vi "Part 2.vi"(11 "Input":string) -> (3 "Output":i64)   [LabVIEW 2021]
uses:
  <vilib>/Utility/miscctls.llb/LVMapReplaceAction.ctl
  2fdae834-c3bc-4fab-b255-983e670ed845.vi
  e0cb1816-1f8c-444e-8856-724e2788fbe8.vi
  <userlib>/_OpenG.lib/string/string.llb/Convert EOLs (String)__ogtk.vi
  <vilib>/Comparison/Equal/Equal Functor/Equal Functor.lvclass
panel:
  out "array":string[](array[string])
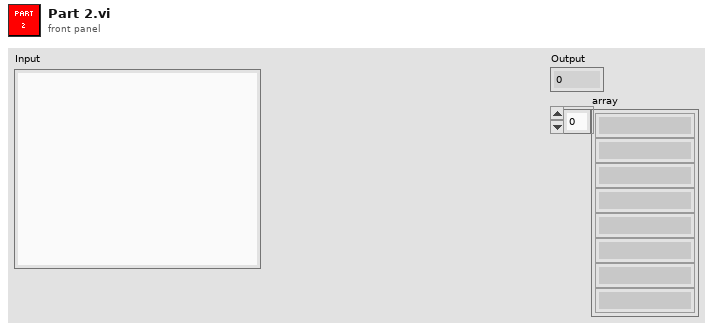
[diagram p1: front panel]
types:
  T1 = map{i32, cluster{"Lens":string[], "Focal Length":i32[]}}
  T2 = typedef "LVMapReplaceAction.ctl" = enum32{"Modify Entry only if found", "Add or Modify Entry", "Delete Entry"}
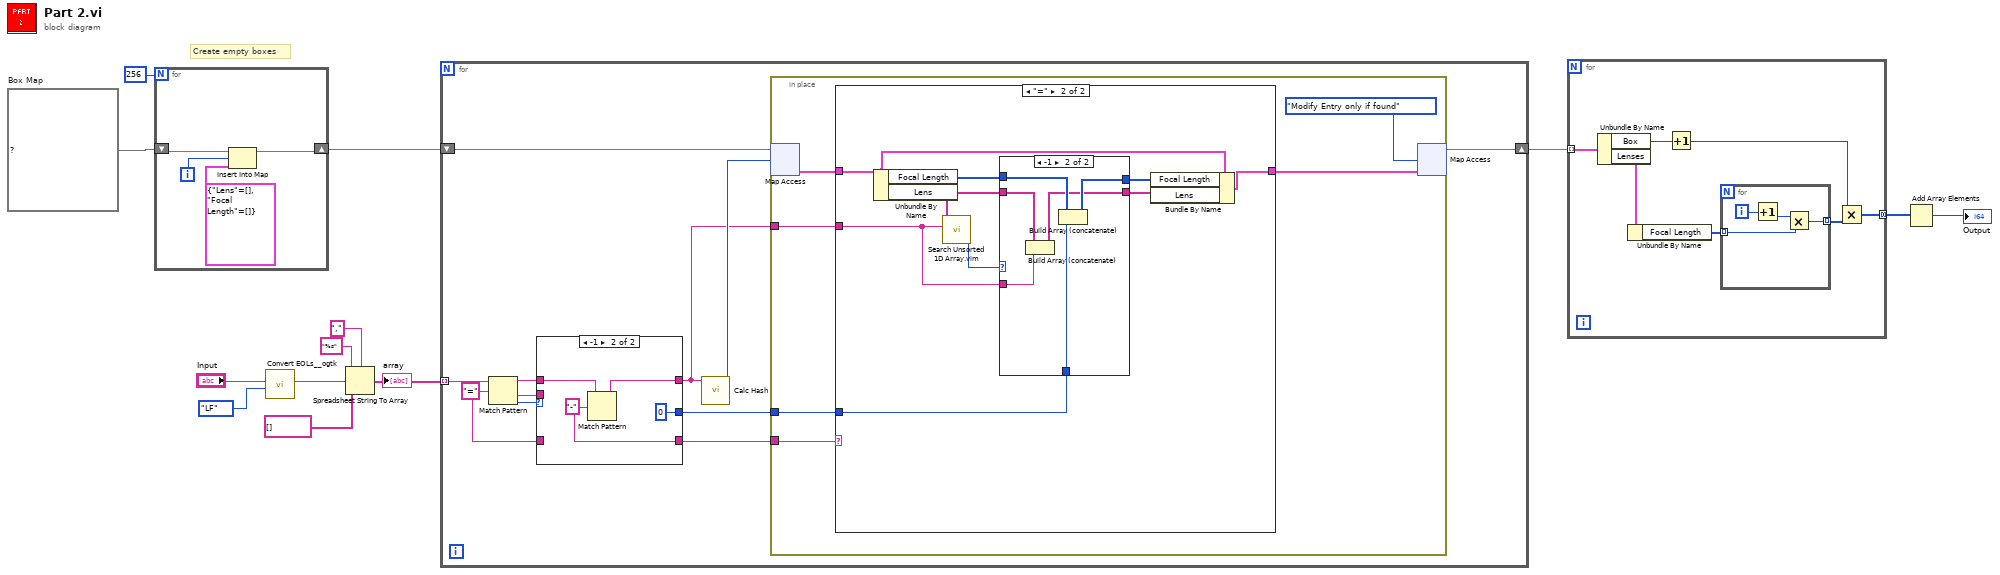
[diagram p0: block diagram]
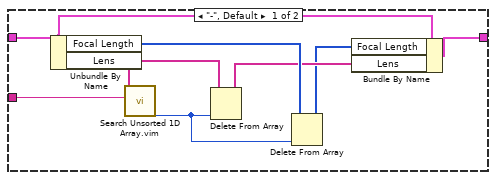
[diagram p2: hidden frame]
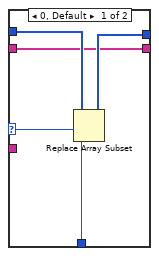
[diagram p3: hidden frame]
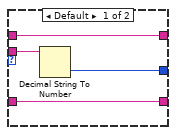
[diagram p4: hidden frame]
diagram:
  w6 = T1 {}  # Box Map
  # "Create empty boxes"
  n1 = for {
    N: 256 -> [_]
    shift-right: [w16] -> w4
    shift-left: w6 -> [w17]
    i -> [w15]
    n2 = Insert Into Map(map in=w17, key=w15, value=cluster{"Lens":string[], "Focal Length":i32[]} {"Lens"=[], "Focal Length"=[]} ("Lenses")) -> (map out=w16:T1)  [unwired: 2 out]
  }
  n3 = call-poly <userlib>:"Convert EOLs__ogtk.vi"("Convert to:"=enum16{"CR", "LF", "CRLF"}."LF", "String in"="Input") -> ("String out"=w9:string)  [unwired: 9 in]
  n4 = Spreadsheet String To Array(delimiter (Tab)=",", format string="%s", spreadsheet string=w9, array type (2D Dbl)=string[] []) -> (array=w7:string[])
  "array" <- w7
  n5 = for {
    tunnel: w7 -> [w28] mode=indexing
    shift-right: [w21] -> w3
    shift-left: w4 -> [w23]
    w25 = "="
    n6 = Match Pattern(string=w28, regular expression=w25) -> (before substring=w24:string, after substring=w26:string, offset past match=w27:i32)  [unwired: 1 in, 1 out]
    n7 = case shown="-1" w27 {
      tunnel: w26 -> [w66 _]
      tunnel: [w65 w68] -> w20
      tunnel: w25 -> [w65 _]
      tunnel: [w64 0] -> w18
      tunnel: w24 -> [w63 w70]
      tunnel: [w63 w69] -> w19
      frame Default {
        n8 = Decimal String To Number(string=w66) -> (number=w64:i32)  [unwired: 2 in, 1 out]
      }
      frame -1 {
        w68 = "-" ("regular expression")
        n9 = Match Pattern(string=w70, regular expression=w68) -> (before substring=w69:string)  [unwired: 1 in, 3 out]
      }
    }
    n10 = call "Calc Hash.vi"("String"=w19) -> ("Numeric"=w22:i32)  [unwired: 10 in]
    n11 = in-place {
      in-place-border: w20 -> [w34]
      in-place-border: w19 -> [w32]
      in-place-border: w18 -> [w29]
      n12 = in-place-map #1(w23, w22) -> (w33:cluster{"Lens":string[], "Focal Length":i32[]})  [unwired: 1 in, 1 out]
      n13 = case shown="\"=\"" w34 {
        tunnel: w33 -> [w38 w50]
        tunnel: w32 -> [w42 w43]
        tunnel: [w35 w48] -> w31
        tunnel: w29 -> [_ w46]
        frame "-", Default {
          n14 = Unbundle By Name(w38) -> ("Focal Length"=w40:i32[], "Lens"=w41:string[])
          n15 = call "Search Unsorted 1D Array.vim"("element"=w42, "unsorted 1D array"=w41) -> ("index of element"=w39:i32)  [unwired: 9 in]
          n16 = Delete From Array(array=w41, index=w39) -> (array with subset deleted=w37:string[])  [unwired: 1 in, 1 out]
          n17 = Delete From Array(array=w40, index=w39) -> (array with subset deleted=w36:i32[])  [unwired: 1 in, 1 out]
          n18 = Bundle By Name(cluster=w38, "Focal Length"=w36, "Lens"=w37) -> (w35:cluster{"Lens":string[], "Focal Length":i32[]})
        }
        frame "=" {
          n19 = Unbundle By Name(w50) -> ("Focal Length"=w51:i32[], "Lens"=w45:string[])
          n20 = call "Search Unsorted 1D Array.vim"("element"=w43, "unsorted 1D array"=w45) -> ("index of element"=w47:i32)  [unwired: 9 in]
          n21 = case shown="-1" w47 {
            selector: w47 -> [w54 _]
            tunnel: w51 -> [w56 w62]
            tunnel: [w55 w61] -> w49
            tunnel: w46 -> [w53 w60]
            tunnel: w45 -> [w52 w59]
            tunnel: [w52 w57] -> w44
            tunnel: w43 -> [_ w58]
            frame 0, Default {
              n22 = Replace Array Subset(array=w56, new element=w53, index=w54) -> (w55:i32[])
            }
            frame -1 {
              n23 = Build Array (concatenate)(w59, w58) -> (w57:string[])
              n24 = Build Array (concatenate)(w62, w60) -> (w61:i32[])
            }
          }
          n25 = Bundle By Name(cluster=w50, "Focal Length"=w49, "Lens"=w44) -> (w48:cluster{"Lens":string[], "Focal Length":i32[]})
        }
      }
      n26 = in-place-map #1(w31, LVMapReplaceAction."Modify Entry only if found" ("action")) -> (w21:T1)  [unwired: 2 out]
    }
  }
  n27 = for {
    tunnel: w3 -> [w77] mode=indexing
    tunnel: [w71] -> w2 mode=concatenating
    n28 = Unbundle By Name(w77) -> ("Box"=w76:i32, "Lenses"=w75:cluster{"Lens":string[], "Focal Length":i32[]})
    n29 = Unbundle By Name(w75) -> ("Focal Length"=w74:i32[])
    n30 = Increment(x=w76) -> (x+1=w72:i32)
    n31 = for {
      tunnel: w74 -> [w79] mode=indexing
      tunnel: [w78] -> w73 mode=indexing
      i -> [w81]
      n32 = Increment(x=w81) -> (x+1=w80:i32)
      n33 = Multiply(x=w80, y=w79) -> (x*y=w78:i32)
    }
    n34 = Multiply(x=w72, y=w73) -> (x*y=w71:i32[])
  }
  n35 = Add Array Elements(numeric array=w2) -> (sum=→"Output":i32)
